vi "SM-s_ NextStatePlus.vi"(7 "Arg Delimiter (:)":string=":", 10 "error?":errorcluster, 11 "States String":string) -> (2 "Argument":string, 3 "Current State":string, 5 "Next States":string)   [LabVIEW 2018]
doc: "<b>State Machine - Next State Plus:</B>\n\nUsed to parse command strings for a string-based State Machine. The \"States String\" holds State Machine commands separated by newlines. Each line has a command/argument for a single iteration of the State Machine. The VI splits the States String into the \"Current State / Argument(s)\" pair and the remaining states left in the \"Next States\" string. The Argument(s) are delimited by a setable delimiter string. The default is a colon \":\". \n\nThe error? input is used to return a command of \"Error Handle\" or optionally an Exit or entire shutdown sequence of commands. This requires external code to pack the error cluster.\n\nAn error code of -9999 is used to invoke and Exit or shutdown sequence, supplied in the source field. EXAMPLE: When used in a timed loop, there is only one iteration available once the loop is aborted, so detect the abort and feed into the error cluster the appropriate command/arg(s) to shutdown gracefully.\n\n2007_12 Mike Ashe\nmichael.ashe@imaginatics.net\nCell: 860-961-0876"
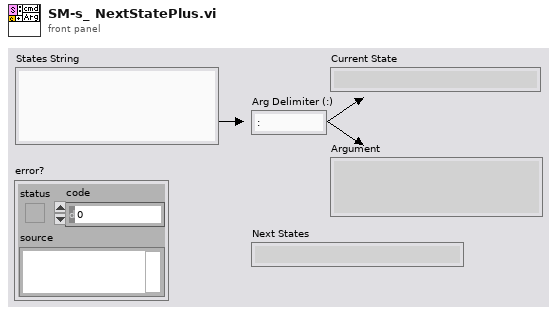
[diagram p1: front panel]
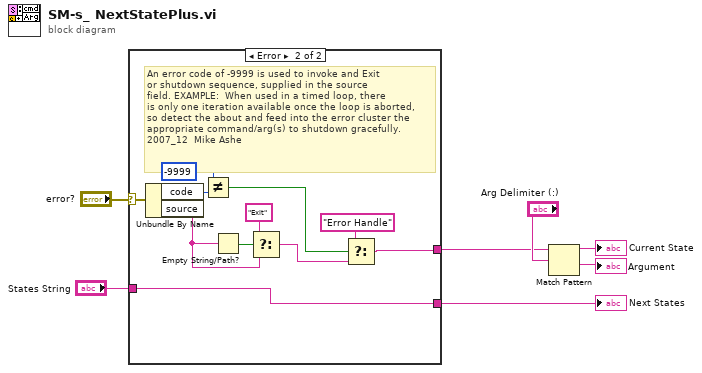
[diagram p0: block diagram]
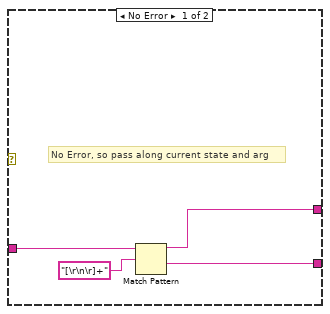
[diagram p2: hidden frame]
diagram:
  n1 = case shown="Error" "error?" {
    selector: "error?" -> [_ w20]
    tunnel: [w10 w21] -> w6
    tunnel: "States String" -> [w11 w12]
    tunnel: [w9 w12] -> w1
    frame No Error {
      # "No Error, so pass along current state and arg"
      n2 = Match Pattern(string=w11, regular expression="[\r\n\r]+" ("Substring")) -> (before substring=w10:string, after substring=w9:string)  [unwired: 1 in, 2 out]
    }
    frame Error {
      # "An error code of -9999 is used to invoke and Exit\nor shutdown sequence, supplied in the source\nfield. EXAMPLE:  When used in a timed loop, there\nis only one iteration available once the loop is aborted,\nso detect the about and feed into the error cluster the\nappropriate command/arg(s) to shutdown gracefully.\n2007_12  Mike Ashe"
      n3 = Unbundle By Name(w20) -> ("code"=w19:i32, "source"=w14:string)
      n4 = Not Equal?(x=-9999, y=w19) -> (x != y?=w17:bool)
      n5 = Empty String/Path?(string/path=w14) -> (empty?=w15:bool)
      n6 = Select(t="Exit", s=w15, f=w14) -> (s? t:f=w13:string)
      n7 = Select(t="Error Handle", s=w17, f=w13) -> (s? t:f=w21:string)
    }
  }
  "Next States" <- w1
  n8 = Match Pattern(string=w6, regular expression="Arg Delimiter (:)") -> (before substring=→"Current State":string, after substring=→"Argument":string)  [unwired: 1 in, 2 out]
